vi "transrotmat (Sub VI).vi"(1 "theta":dbl) -> (0 "J":dbl[][](array[numeric]))   [LabVIEW 2011]
uses:
  <vilib>/imath/engines/lvmath2/RunTimeEngine/NodeEndStatement/NIMS_NodeEndStatement_Output.vi
  <instcachedir>/0/NIMS_NodeEndStatement_Output_53EC0D466D134D7ABD903AC30B43404B.lvgen/NIMS_NodeEndStatement_Output_53EC0D466D134D7ABD903AC30B43404B_002.vi
  <vilib>/imath/engines/lvmath2/RunTimeEngine/ErrorHandling/NIMS_Finalize Error.vi
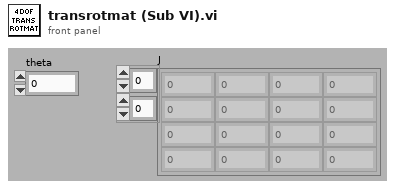
[diagram p1: front panel]
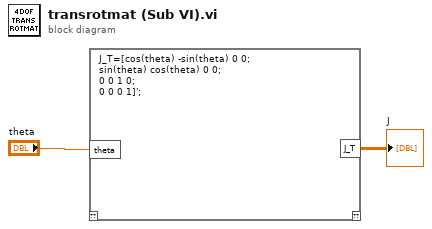
[diagram p0: block diagram]
diagram:
  n1 = mathscript code="J_T=[cos(theta) -sin(theta) 0 0;\nsin(theta) cos(theta) 0 0;\n0 0 1 0;\n0 0 0 1]';"("theta"="theta") -> ("J_T"=→"J":dbl[][])  [unwired: 1 in, 1 out]
